vi "ELVIS III v1.0 Close DO Block.vi"(8 "error in (no error)":errorcluster, 10 "DO (N Samples) Channel List":T3, 11 "myRIO Ref In":T1) -> (0 "error out":errorcluster)   [LabVIEW 2021]
uses:
  <vilib>/myRIO/Common/Instrument Driver Framework/myRIO v1.0/DO Block/typedefs/DO Block Channels List.ctl
  <vilib>/myRIO/Common/Instrument Driver Framework/myRIO v1.0/DO Block/typedefs/DO Block Channels Enum.ctl
  <vilib>/myRIO/Common/Instrument Driver Framework/Utilities/typedefs/myRIO v1.0 Reference.ctl
  <vilib>/myRIO/Common/Instrument Driver Framework/Utilities/typedefs/Generic FPGA Reference.ctl
  <vilib>/myRIO/Common/Instrument Driver Framework/Utilities/vis/Sample Rate To Ticks.vi
  <vilib>/myRIO/Common/Instrument Driver Framework/ELVIS III v1.0/DO Block/vis/ELVIS III v1.0 Build MUX Configuration DO Block.vi
  <vilib>/myRIO/Common/Instrument Driver Framework/ELVIS III v1.0/Resource Manager/vis/ELVIS III v1.0 Create Configuration List.vi
  <vilib>/myRIO/Common/Instrument Driver Framework/myRIO v1.0/Resource Manager/vis/myRIO v1.0 Block Write Configuration.vi
  <vilib>/myRIO/Common/Instrument Driver Framework/ELVIS III v1.0/DO Block/vis/ELVIS III v1.0 DO Build Bank Data.vi
  <vilib>/myRIO/Common/Instrument Driver Framework/ELVIS III v1.0/DO Block/vis/ELVIS III v1.0 DO Enqueue Data.vi
  <vilib>/myRIO/Common/Instrument Driver Framework/ELVIS III v1.0/Resource Manager/vis/ELVIS III v1.0 Configure IO.vi
  <vilib>/myRIO/Common/Instrument Driver Framework/ELVIS III v1.0/Resource Manager/vis/ELVIS III v1.0 Configure DO DIR.vi
  <vilib>/myRIO/Common/Instrument Driver Framework/ELVIS III v1.0/Resource Manager/vis/ELVIS III v1.0 Unreserve Channel List.vi
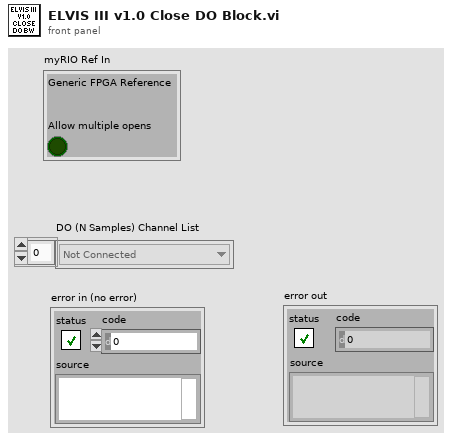
[diagram p1: front panel]
types:
  T1 = typedef "myRIO v1.0 Reference.ctl" = cluster{"Generic FPGA Reference":T2, "Allow multiple opens":bool}
  T2 = typedef "Generic FPGA Reference.ctl" = refnum<k20>
  T3 = typedef "DO Block Channels List.ctl" = T4[]
  T4 = typedef "DO Block Channels Enum.ctl" = enum16{"Not Connected", "A/DO0 (N Samples)", "A/DO1 (N Samples)", "A/DO2 (N Samples)", "A/DO3 (N Samples)", "A/DO4 (N Samples)", "A/DO5 (N Samples)", "A/DO6 (N Samples)", "A/DO7 (N Samples)", "A/DO8 (N Samples)", "A/DO9 (N Samples)", "A/DO10 (N Samples)", "A/DO11 (N Samples)", "A/DO12 (N Samples)", "A/DO13 (N Samples)", "A/DO14 (N Samples)", "A/DO15 (N Samples)", "A/DO16 (N Samples)", "A/DO17 (N Samples)", "A/DO18 (N Samples)", "A/DO19 (N Samples)", "B/DO0 (N Samples)", "B/DO1 (N Samples)", "B/DO2 (N Samples)", "B/DO3 (N Samples)", "B/DO4 (N Samples)", "B/DO5 (N Samples)", "B/DO6 (N Samples)", "B/DO7 (N Samples)", "B/DO8 (N Samples)", "B/DO9 (N Samples)", "B/DO10 (N Samples)", "B/DO11 (N Samples)", "B/DO12 (N Samples)", "B/DO13 (N Samples)", "B/DO14 (N Samples)", "B/DO15 (N Samples)", "B/DO16 (N Samples)", "B/DO17 (N Samples)", "B/DO18 (N Samples)", "B/DO19 (N Samples)"}
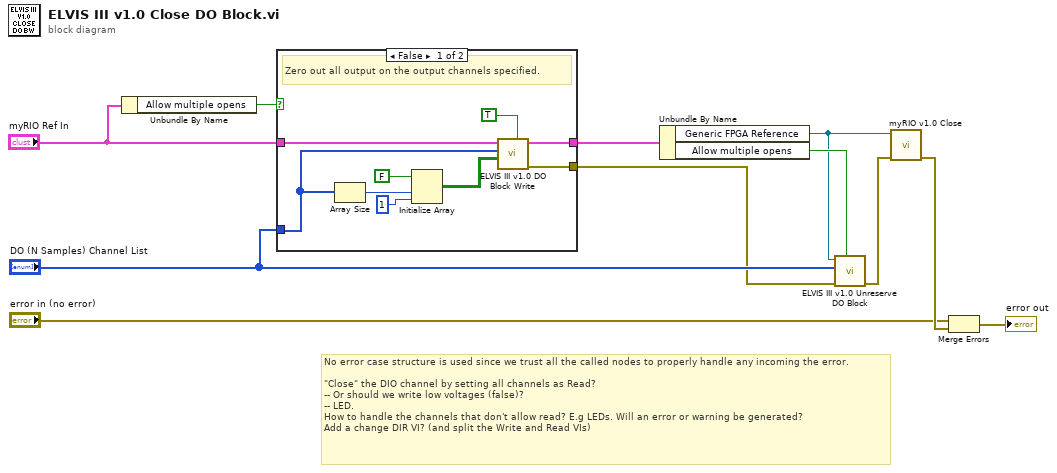
[diagram p0: block diagram]
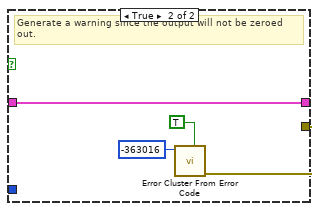
[diagram p2: hidden frame]
diagram:
  # "No error case structure is used since we trust all the called nodes to properly handle any incoming the error.\n\n\"Close\" the DIO channel by setting all channels as Read?\n-- Or should we write low voltages (false)?\n-- LED.\nHow to handle the channels that don't allow read? E.g LEDs. Will an error or warning be generated?\nAdd a change DIR VI? (and split the Write and Read VIs)"
  n1 = Unbundle By Name("myRIO Ref In") -> ("Allow multiple opens"=w7:bool)
  n2 = case shown="False" w7 {
    tunnel: "myRIO Ref In" -> [w20 w24]
    tunnel: [w14 w24] -> w3
    tunnel: "DO (N Samples) Channel List" -> [w19 _]
    tunnel: [w13 w21] -> w1
    frame False {
      # "Zero out all output on the output channels specified."
      n3 = Array Size(array=w19) -> (size(s)=w16:i32)
      n4 = Initialize Array(FALSE, w16, 1 ("dimension size")) -> (w17:bool[][])
      n5 = call <vilib>:"ELVIS III v1.0 DO Block Write.vi"("Wait Until Done?"=TRUE, "Data by Channel"=w17, "DO (N Samples) Channel List"=w19, "myRIO Ref In"=w20) -> ("error out"=w13:errorcluster, "myRIO Ref Out"=w14:T1)  [unwired: 6 in]
    }
    frame True {
      # "Generate a warning since the output will not be zeroed out."
      n6 = call <vilib>:"Error Cluster From Error Code.vi"("is warning? (False)"=TRUE, "error code (0)"=-363016) -> ("error out"=w21:errorcluster)  [unwired: 7 in]
    }
  }
  n7 = Unbundle By Name(w3) -> ("Generic FPGA Reference"=w2:T2, "Allow multiple opens"=w9:bool)
  n8 = call <vilib>:"ELVIS III v1.0 Unreserve DO Block.vi"("Allow multiple opens?"=w9, "error in (no error)"=w1, "DO (N Samples) Channel List"="DO (N Samples) Channel List", "Generic FPGA Reference"=w2) -> ("error out"=w11:errorcluster)  [unwired: 7 in]
  n9 = call <vilib>:"myRIO v1.0 Close.vi"("error in (no error)"=w11, "myRIO FPGA Ref In"=w2) -> ("error out"=w10:errorcluster)  [unwired: 9 in]
  n10 = Merge Errors("error in (no error)", w10) -> (→"error out":errorcluster)
